vi "error.vi"(5 "Iteration duration":u32, 7 "stop":bool, 8 "idx":i32, 11 "Qube":refnum<class "System.lvclass">) -> (0 "abort?":bool, 3 "Qube":refnum<class "System.lvclass">)   [LabVIEW 2021, in "System.lvclass"]
uses:
  System.lvclass
  System.lvclass/System.ctl
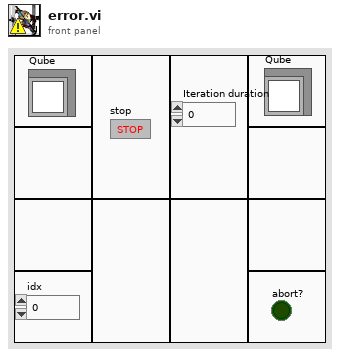
[diagram p1: front panel]
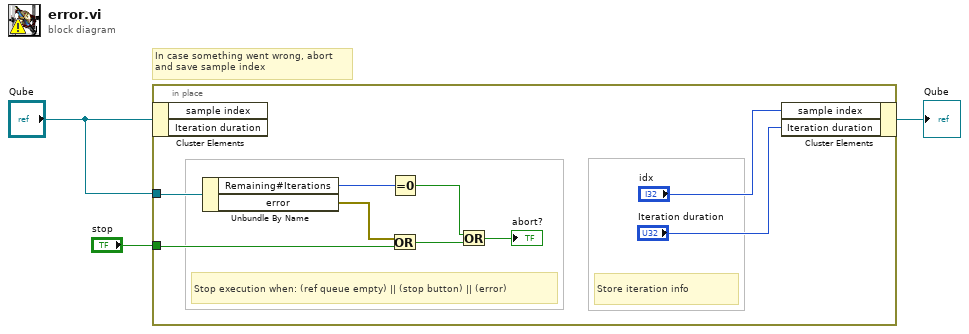
[diagram p0: block diagram]
diagram:
  # "In case something went wrong, abort\nand save sample index"
  n1 = in-place {
    in-place-border: "stop" -> [w12]
    in-place-border: "Qube" -> [w4]
    # "Store iteration info"
    # "Stop execution when: (ref queue empty) || (stop button) || (error)"
    n2 = in-place-cluster #1("Qube") -> ()  [unwired: 2 out]
    n3 = Unbundle By Name(w4) -> ("Remaining#Iterations"=w7:u32, "error"=w10:errorcluster)
    n4 = Equal To 0?(x=w7) -> (x = 0?=w6:bool)
    n5 = Or(x=w10, y=w12) -> (x .or. y?=w11:bool)
    n6 = Or(x=w6, y=w11) -> (x .or. y?=→"abort?":bool)
    n7 = in-place-cluster #1("sample index"="idx", "Iteration duration"="Iteration duration") -> (→"Qube":refnum<class "System.lvclass">)
  }
